vi "FindActiveDevice.vi"() -> (0 "error out":errorcluster, 3 "task out":refnum<k21>)   [LabVIEW 2013, in "main.lvlib"]
uses:
  main.lvlib
  <vilib>/DAQmx/create/channels.llb/DAQmx Create Channel (AI-Voltage-Basic).vi
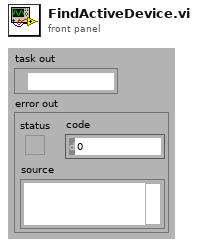
[diagram p1: front panel]
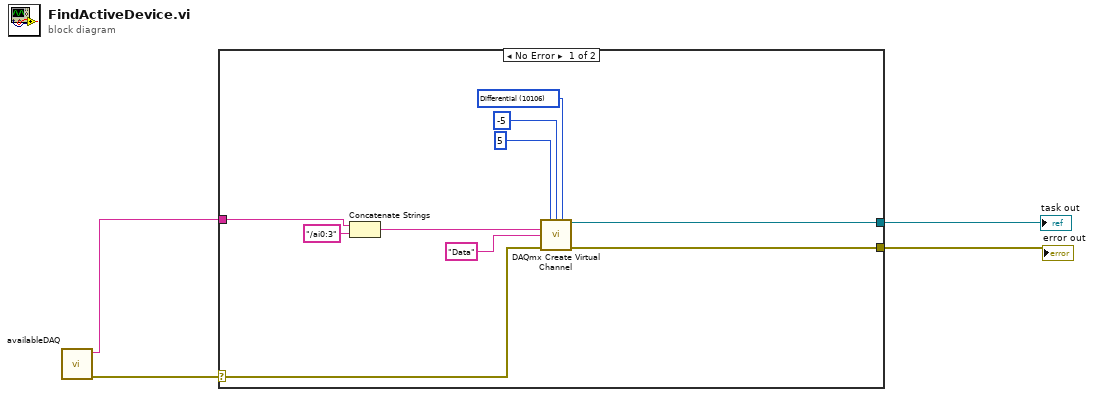
[diagram p0: block diagram]
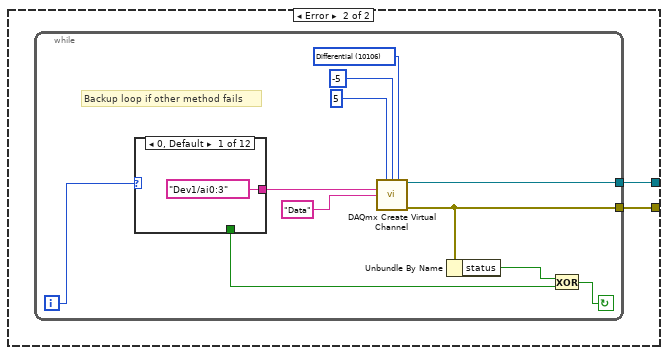
[diagram p2: hidden frame]
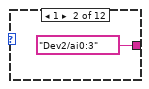
[diagram p3: hidden frame]
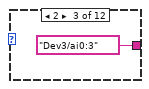
[diagram p4: hidden frame]
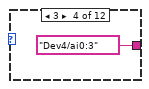
[diagram p5: hidden frame]
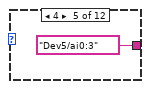
[diagram p6: hidden frame]
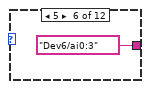
[diagram p7: hidden frame]
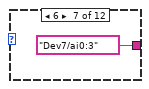
[diagram p8: hidden frame]
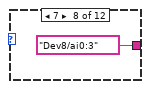
[diagram p9: hidden frame]
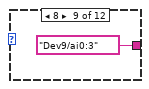
[diagram p10: hidden frame]
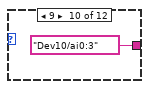
[diagram p11: hidden frame]
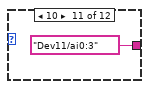
[diagram p12: hidden frame]
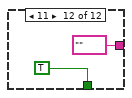
[diagram p13: hidden frame]
diagram:
  n1 = call "availableDAQ.vi"() -> ("error out"=w2:errorcluster, "DAQmx Device Name"=w1:tag)  [unwired: 10 in]
  n2 = case shown="No Error" w2 {
    selector: w2 -> [w9 _]
    tunnel: [w5 w16] -> w4
    tunnel: [w10 w15] -> w3
    tunnel: w1 -> [w6 _]
    frame No Error {
      w11 = 10106 items=["default"=-1, "RSE"=10083, "NRSE"=10078, "Differential"=10106, "Pseudodifferential"=12529] ("input terminal configuration")
      n3 = Concatenate Strings(w6, "/ai0:3" ("string")) -> (w8:string)
      n4 = call-poly <vilib>:"DAQmx Create Virtual Channel.vi"("maximum value"=5, "minimum value"=-5, "input terminal configuration"=w11, "physical channels"=w8, "name to assign"="Data", "error in"=w9) -> ("task out"=w5:refnum<k21>, "error out"=w10:errorcluster)  [unwired: 8 in]
    }
    frame Error {
      n5 = while {
        tunnel: [w18] -> w16
        tunnel: [w17] -> w15
        i -> [w22]
        stop <- w21 continue-if-true
        w24 = 10106 items=["default"=-1, "RSE"=10083, "NRSE"=10078, "Differential"=10106, "Pseudodifferential"=12529] ("input terminal configuration")
        # "Backup loop if other method fails"
        n6 = case shown="0, Default" w22 {
          tunnel: [tag "Dev1/ai0:3" ("physical channels") tag "Dev2/ai0:3" ("physical channels") tag "Dev3/ai0:3" ("physical channels") tag "Dev4/ai0:3" ("physical channels") tag "Dev5/ai0:3" ("physical channels") tag "Dev6/ai0:3" ("physical channels") tag "Dev7/ai0:3" ("physical channels") tag "Dev8/ai0:3" ("physical channels") tag "Dev9/ai0:3" ("physical channels") tag "Dev10/ai0:3" ("physical channels") tag "Dev11/ai0:3" ("physical channels") tag "" ("physical channels")] -> w23
          tunnel: [_ _ _ _ _ _ _ _ _ _ _ TRUE] -> w19
          frame 0, Default {
          }
          frame 1 {
          }
          frame 2 {
          }
          frame 3 {
          }
          frame 4 {
          }
          frame 5 {
          }
          frame 6 {
          }
          frame 7 {
          }
          frame 8 {
          }
          frame 9 {
          }
          frame 10 {
          }
          frame 11 {
          }
        }
        n7 = call-poly <vilib>:"DAQmx Create Virtual Channel.vi"("maximum value"=5, "minimum value"=-5, "input terminal configuration"=w24, "physical channels"=w23, "name to assign"="Data") -> ("task out"=w18:refnum<k21>, "error out"=w17:errorcluster)  [unwired: 9 in]
        n8 = Unbundle By Name(w17) -> ("status"=w20:bool)
        n9 = Exclusive Or(1:w19, 2:w20) -> (0:w21:bool)
      }
    }
  }
  "task out" <- w4
  "error out" <- w3
